vi "play-z-scope.vi"() -> ()   [LabVIEW 2017]
uses:
  <vilib>/userdefined/High Color/nirio_resource_hc.ctl
  <vilib>/FPGAPlugInAG/cRIO-9082/niLvFpga_Open_cRIO-9082.vi
  <vilib>/rvi/interface/common/dynamic/niFpgaDynamicAddResources.vi
  <vilib>/FPGAPlugInAG/Dynamic/niLvFpga_Reset_Dynamic.vi
  <vilib>/rvi/interface/common/niFpgaWaitOnOcc.vi
  <vilib>/Utility/error.llb/Error Cluster From Error Code.vi
  <vilib>/rvi/errors/niLvFpgaAdjustHostInterfaceError.vi
  <vilib>/FPGAPlugInAG/Dynamic/niLvFpga_Run_Dynamic.vi
  <vilib>/Utility/file.llb/Write Delimited Spreadsheet (DBL).vi
  <vilib>/FPGAPlugInAG/Dynamic/niLvFpga_Close_Dynamic.vi
  <vilib>/rvi/interface/nirviOpenFPGA/nirviOpenFPGA.xnode
  FPGA Bitfiles/afmimagingcontro_FPGATargetSPARTA_z-scope_kJamH4E+AOg.lvbitx
  <vilib>/rvi/interface/nirviMethod/nirviMethod.xnode
  <vilib>/rvi/interface/nirviReadWriteControl/nirviReadWriteControl.xnode
  <vilib>/rvi/interface/nirviCloseFPGA/nirviCloseFPGA.xnode
  <vilib>/rvi/errors/niLvFpgaMergeErrorWithErrorCode.vi
  <vilib>/rvi/interface/Simulation/niFpgaSimulationCallBeginRW.vi
  <vilib>/FPGAPlugInAG/Dynamic/niLvFpga_ReadFifo_Dynamic.vi
  NiFpgaLv.dll
  controls/expMetaData.ctl
  <userlib>/_matio/level5.lvlib
  <vilib>/FPGAPlugInAG/Dynamic/niLvFpga_ConfigureFifo_Dynamic.vi
  <userlib>/_matio/level5/Public/Write/Append Data Element.llb/Append Data Element (Anything).vi
panel:
  out "boolean  indicators":T1
  out "Waveform Chart":dbl[](graph)
  in  "sysID_Z_axis_params":T2={"TOL"=0.3, "ramp-rate"=-5e-05, "z-u-max"=0.0, "offset"=0.0, "Ki"=0.005, "Z-error-threshold"=0.05, "Z-settled-samples\nthreshold "=0, "z_UP"=0.0, "zup-N"=0}
  out "result string":string
  in  "Tab Control":enum32{"Main Settings", "Host Debug"}(tab)
  in  "outputData":path=path "Z:/afm-cs/z-scope/data-out_tmp.csv"
  in  "TsTicks":u32=1600
  out "iter":i32
  in  "ABORT":bool
  in  "Ki-xy":sgl
  in  "xy-bound":sgl=1.0
  out "y iter":i32
  out "z-control":dbl[](graph)
  out "z-error":dbl[](graph)
  # "- If collect all = fasle and collect move = false,\nwe only collect measurement data.\n- If collect all = false, and collect move = true,\nwe collect measurement and move data.\n- If collect all = true, we collect everything."
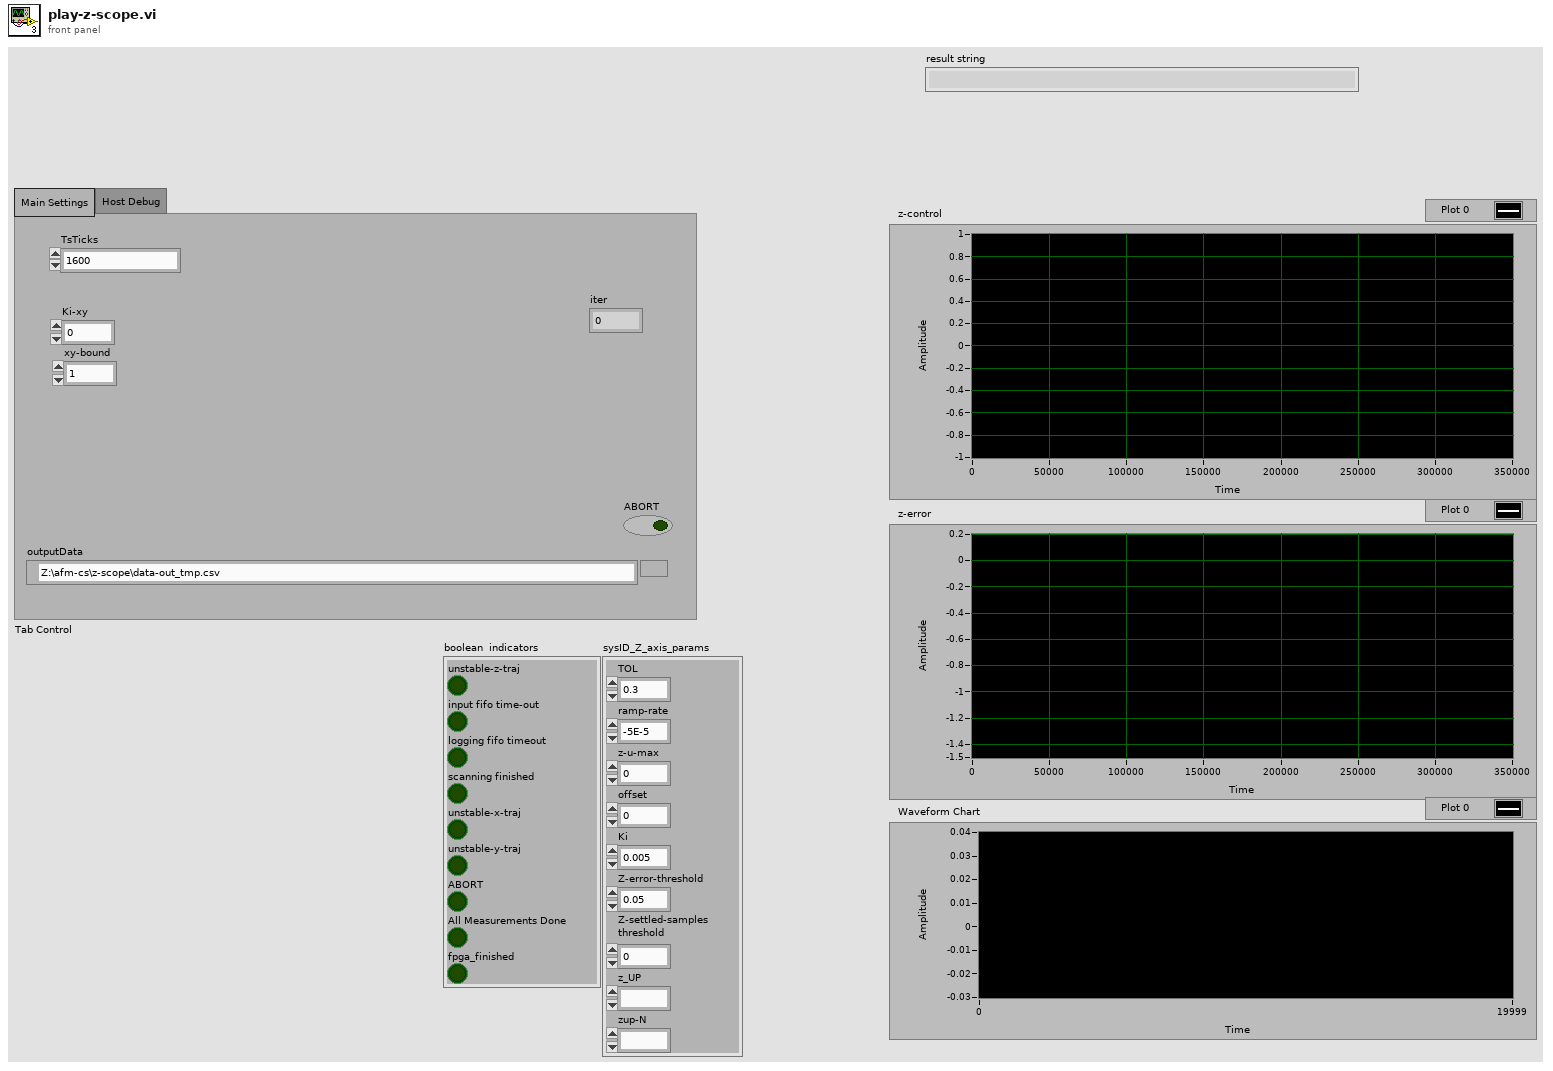
[diagram p1: front panel]
types:
  T1 = cluster{"unstable-z-traj":bool, "input fifo time-out":bool, "logging fifo timeout":bool, "scanning finished":bool, "unstable-x-traj":bool, "unstable-y-traj":bool, "ABORT":bool, "All Measurements Done":bool, "fpga_finished":bool}
  T2 = cluster{"TOL":sgl, "ramp-rate":sgl, "z-u-max":sgl, "offset":sgl, "Ki":sgl, "Z-error-threshold":sgl, "Z-settled-samples\nthreshold ":i16, "z_UP":fxp<+/-,16,5>, "zup-N":i16}
  T3 = typedef "nirio_resource_hc.ctl" = tag
  T4 = enum16{"open", "replace", "create", "open or create", "replace or create", "replace or create with confirmation"}
  T5 = typedef "expMetaData.ctl" = cluster{"xy_error_threshold":sgl, "xy_settled_samples_threshold":i16, "Ki_xy":sgl, "state_counts":dbl[], "TOL":sgl, "ramp_rate":sgl, "z_u_max":sgl, "setpoint":sgl, "Ki":sgl, "Z_error_threshold":sgl, "Z_settled_samples_threshold ":i16, "z_UP":sgl, "zup_N":i16, "Num":sgl[], "Den":sgl[], "max_Z_settle_samples":i16, "Kiz_down":sgl, "do_xy_CL":bool, "do_Alt_Ztrigger":bool, "output-data-path":path, "input-data-path":path, "uz_safe":sgl, "zup_rate":sgl}
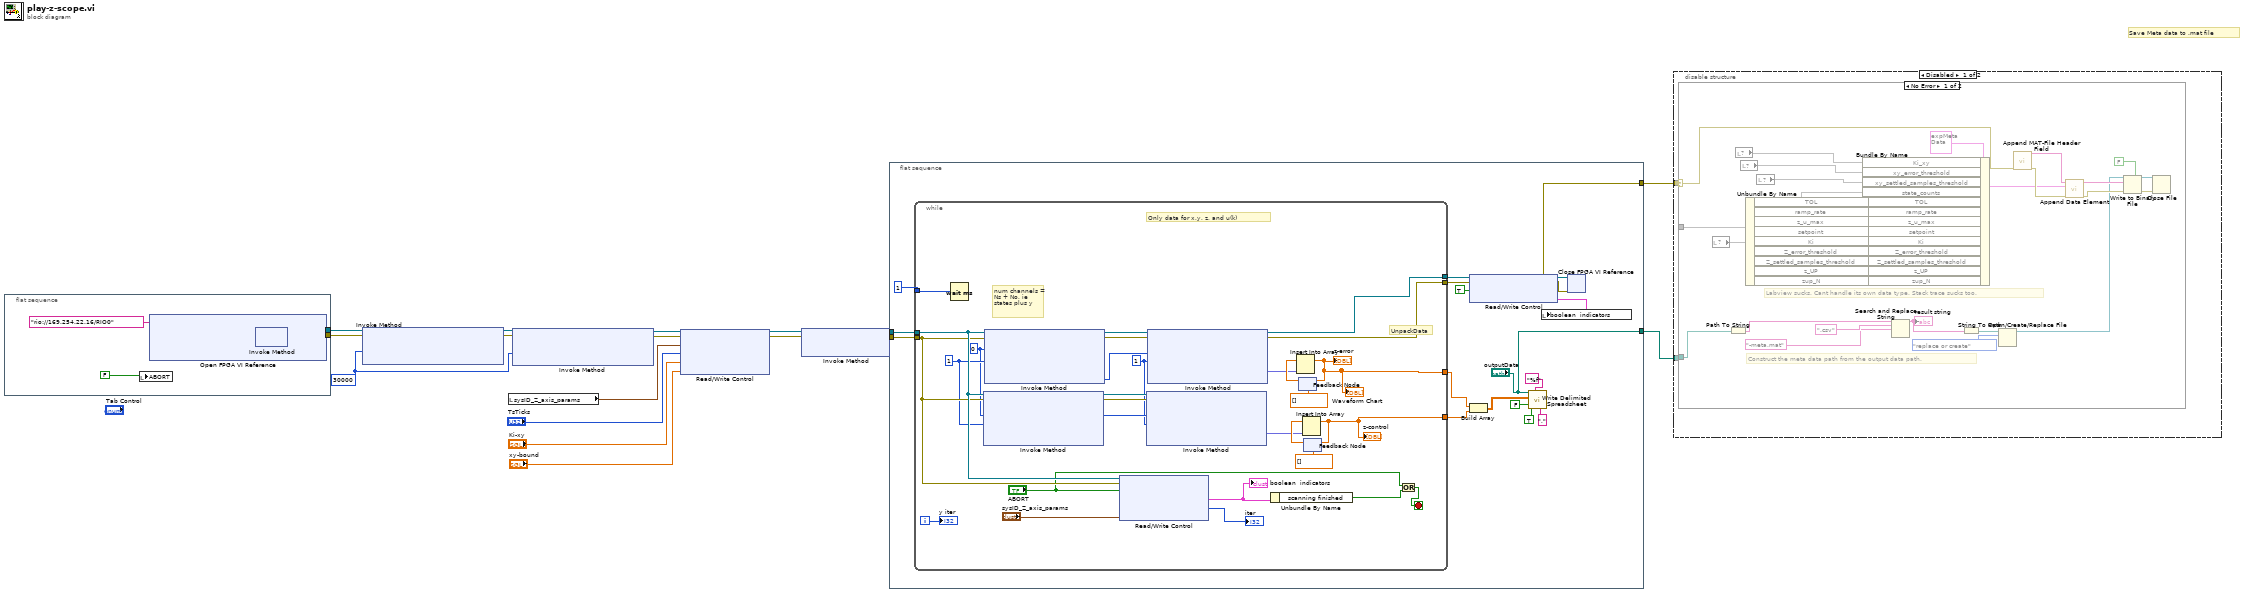
[diagram p0: block diagram]
diagram:
  w4 = 30000
  # "Save Meta data to .mat file"
  n1 = flat-sequence {
    tunnel: [w20] -> w17
    tunnel: [w19] -> w16
    frame #0 {
      n2 = local write "ABORT"(FALSE) -> ()
      n3 = xnode "Open FPGA VI Reference"("resource name"=T3 "rio://169.254.22.16/RIO0") -> ("FPGA VI Reference Out"=w23:refnum<k20>, "error out"=w22:errorcluster)  [unwired: 1 in]
      n4 = xnode "Invoke Method"("FPGA VI Reference In"=w23, "error in"=w22) -> ("FPGA VI Reference Out"=w20:refnum<k20>, "error out"=w19:errorcluster)
    }
  }
  n5 = xnode "Invoke Method"("FPGA VI Reference In"=w17, "error in"=w16, "Requested Depth"=w4) -> ("FPGA VI Reference Out"=w8:refnum<k20>, "error out"=w7:errorcluster)  [unwired: 1 out]
  n6 = local read "sysID_Z_axis_params"() -> (w3:T2)
  n7 = xnode "Invoke Method"("FPGA VI Reference In"=w8, "error in"=w7, "Requested Depth"=w4) -> ("FPGA VI Reference Out"=w6:refnum<k20>, "error out"=w5:errorcluster)  [unwired: 1 out]
  n8 = xnode "Read/Write Control"("FPGA VI Reference In"=w6, "error in"=w5, "sysID_Z_axis_params"=w3, "TsTicks"="TsTicks", "Ki-xy"="Ki-xy", "xy-bound"="xy-bound") -> ("FPGA VI Reference Out"=w10:refnum<k20>, "error out"=w9:errorcluster)
  n9 = xnode "Invoke Method"("FPGA VI Reference In"=w10, "error in"=w9) -> ("FPGA VI Reference Out"=w12:refnum<k20>, "error out"=w11:errorcluster)  [unwired: 1 in]
  n10 = flat-sequence {
    tunnel: w11 -> [w39]
    tunnel: w12 -> [w30]
    tunnel: [w28] -> w13
    tunnel: ["outputData"] -> w14
    frame #0 {
      n11 = while {
        tunnel: 1 -> [w69]
        tunnel: w30 -> [w54]
        tunnel: w39 -> [w53]
        tunnel: [w59] -> w34
        tunnel: [w62] -> w33
        tunnel: [w44] -> w25
        tunnel: [w41] -> w26
        i -> [w66]
        stop <- w65 stop-if-true
        w46 = 1
        w45 = 0 ("Timeout (ms)")
        w47 = 1 ("Timeout (ms)")
        # "num channels = Ns + No, ie states plus y"
        # "Only data for x,y, z, and u(k)"
        # "UnpackData"
        n12 = Wait (ms)(milliseconds to wait=w69) -> ()  [unwired: 1 out]
        n13 = xnode "Invoke Method"("FPGA VI Reference In"=w54, "error in"=w53, "Number of Elements"=w45, "Timeout (ms)"=w47) -> ("FPGA VI Reference Out"=w56:refnum<k20>, "error out"=w55:errorcluster, "Elements Remaining"=w57:u32)  [unwired: 1 out]
        n14 = xnode "Invoke Method"("FPGA VI Reference In"=w54, "error in"=w53, "Number of Elements"=w45, "Timeout (ms)"=w47) -> ("FPGA VI Reference Out"=w67:refnum<k20>, "error out"=w68:errorcluster, "Elements Remaining"=w43:u32)  [unwired: 1 out]
        n15 = xnode "Read/Write Control"("FPGA VI Reference In"=w54, "error in"=w53, "ABORT"="ABORT", "sysID_Z_axis_params"="sysID_Z_axis_params") -> ("boolean  indicators"=w42:T1, "iter"=→"iter":i32)  [unwired: 2 out]
        "boolean  indicators" <- w42
        n16 = xnode "Invoke Method"("FPGA VI Reference In"=w56, "error in"=w55, "Number of Elements"=w57, "Timeout (ms)"=w46) -> ("Data"=w50:fxp<+/-,16,5>[])  [unwired: 3 out]
        n17 = xnode "Invoke Method"("FPGA VI Reference In"=w67, "error in"=w68, "Number of Elements"=w43, "Timeout (ms)"=w46) -> ("FPGA VI Reference Out"=w59:refnum<k20>, "error out"=w62:errorcluster, "Data"=w58:fxp<+/-,16,5>[])  [unwired: 1 out]
        n18 = Unbundle By Name(w42) -> ("scanning finished"=w61:bool)
        n19 = feedback #1(dbl[] []) -> (w63:dbl[])
        n20 = Insert Into Array(array=w63, new element=w58) -> (w44:dbl[])  [unwired: 1 in]
        "z-error" <- w44
        "Waveform Chart" <- w44
        n21 = feedback-in #1(w44) -> ()
        n22 = feedback #2(dbl[] []) -> (w51:dbl[])
        n23 = Insert Into Array(array=w51, new element=w50) -> (w41:dbl[])  [unwired: 1 in]
        "z-control" <- w41
        n24 = feedback-in #2(w41) -> ()
        n25 = Or(x="ABORT", y=w61) -> (x .or. y?=w65:bool)
        "y iter" <- w66
      }
      n26 = Build Array(w25, w26) -> (w24:dbl[][])
      n27 = xnode "Read/Write Control"("FPGA VI Reference In"=w34, "error in"=w33, "ABORT"=TRUE) -> ("FPGA VI Reference Out"=w31:refnum<k20>, "error out"=w28:errorcluster, "boolean  indicators"=w27:T1)
      n28 = call-poly <vilib>:"Write Delimited Spreadsheet.vi"("file path (dialog if empty)"="outputData", "format (%.3f)"="%f", "2D data"=w24, "append to file? (new file:F)"=FALSE, "transpose? (no:F)"=TRUE, "delimiter (\\t)"=",") -> ()  [unwired: 8 in, 2 out]
      n29 = local write "boolean  indicators"(w27) -> ()
      n30 = xnode "Close FPGA VI Reference"("FPGA VI Reference In"=w31, "error in"=w28) -> ()  [unwired: 1 out]
    }
  }
  n31 = disable-structure shown="Disabled" {
    disable-tunnel: w14 -> [w71 _]
    disable-tunnel: w13 -> [w70 _]
    frame Disabled {
      n32 = case shown="No Error" w70 {
        selector: w70 -> [w92 _]
        tunnel: w71 -> [w73 _]
        tunnel: _ -> [w78 _]
        frame No Error {
          # "Construct the meta data path from the output data path."
          # "Labview sucks. Cant handle its own data type. Stack trace sucks too."
          n33 = local read item#-1() -> (w77)
          n34 = Path To String(path=w73) -> (string=w95:string)
          n35 = local read item#-1() -> (w76)
          n36 = local read item#-1() -> (w75)
          n37 = Unbundle By Name(w77) -> ("TOL"=w88, "ramp_rate"=w87, "z_u_max"=w86, "setpoint"=w85, "Ki"=w84, "Z_error_threshold"=w83, "Z_settled_samples_threshold"=w82, "z_UP"=w81, "zup_N"=w80)
          n38 = local read item#-1() -> (w74)
          n39 = Bundle By Name(cluster=T5 {"xy_error_threshold"=0.1, "xy_settled_samples_threshold"=200, "Ki_xy"=0.005, "state_counts"=[], "TOL"=0.3, "ramp_rate"=-5e-06, "z_u_max"=5.0, "setpoint"=0.0, "Ki"=0.001, "Z_error_threshold"=0.0, "Z_settled_samples_threshold "=0, "z_UP"=1.5, "zup_N"=5000, "Num"=[-0.00254, 0.000408, 0.00295, 0.0, 0.0, 0.0, 0.0, 0.0, 0.0], "Den"=[0.982758, -1.98194, 1.0, 0.0, 0.0, 0.0, 0.0, 0.0, 0.0], "max_Z_settle_samples"=5000, "Kiz_down"=0.001, "do_xy_CL"=FALSE, "do_Alt_Ztrigger"=FALSE, "output-data-path"=path "", "input-data-path"=path "", "uz_safe"=0.0, "zup_rate"=0.0} ("ExpMetaData"), "Ki_xy"=w76, "xy_error_threshold"=w75, "xy_settled_samples_threshold"=w74, "state_counts"=w78, "TOL"=w88, "ramp_rate"=w87, "z_u_max"=w86, "setpoint"=w85, "Ki"=w84, "Z_error_threshold"=w83, "Z_settled_samples_threshold"=w82, "z_UP"=w81, "zup_N"=w80) -> (w89:T5)
          n40 = Search and Replace String(input string=w95, search string=".csv", replace string="-meta.mat" ("replace string (\"\")")) -> (result string=w94:string)  [unwired: 5 in, 3 out]
          "result string" <- w94
          n41 = String To Path(string=w94) -> (path=w91:path)
          n42 = Open/Create/Replace File(file path (use dialog)=w91, operation (0:open)=T4."replace or create") -> (refnum out=w90:refnum<file>)  [unwired: 4 in, 2 out]
          n43 = call <userlib>:"Append MAT-File Header Field.vi"("error"=w92) -> ("result string"=w103:string, "error out"=w93:errorcluster)  [unwired: 13 in]
          n44 = call-poly <userlib>:"Append Data Element.vi"("initial string"=w103, "data"=w89, "error in (no error)"=w93) -> ("result string"=w101:string, "error out"=w102:errorcluster)  [unwired: 11 in]
          n45 = Write to Binary File(file (use dialog)=w90, data=w101, error in=w102, 5:FALSE ("prepend array or string size? (T)")) -> (refnum out=w98:refnum<file>, error out=w99:errorcluster)  [unwired: 2 in, 1 out]
          n46 = Close File(refnum=w98, error in=w99) -> ()  [unwired: 2 out]
        }
        frame Error {
        }
      }
    }
    frame Enabled {
    }
  }
